vi "Min Max Abs.vi"(2 "b":dbl, 3 "a":dbl) -> (0 "MaxAbs(a,b)":dbl, 1 "MinAbs(a,b)":dbl)   [LabVIEW 2016]
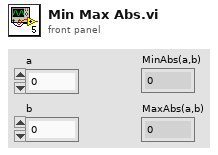
[diagram p1: front panel]
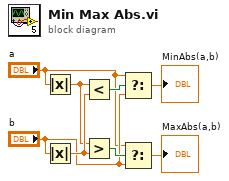
[diagram p0: block diagram]
diagram:
  n1 = Absolute Value(x="a") -> (abs(x)=w2:dbl)
  n2 = Absolute Value(x="b") -> (abs(x)=w7:dbl)
  n3 = Less?(x=w2, y=w7) -> (x < y?=w8:bool)
  n4 = Greater?(x=w2, y=w7) -> (0:w6:bool)
  n5 = Select(t="a", s=w8, f="b") -> (s? t:f=→"MinAbs(a,b)":dbl)
  n6 = Select(t="a", s=w6, f="b") -> (s? t:f=→"MaxAbs(a,b)":dbl)
